vi "Rotate Point.vi"(6 "Para":cluster{"Absolute?":bool, "Angle":dbl}={"Absolute?"=TRUE, "Angle"=0.0}, 8 "错误输入":errorcluster, 10 "Center":T1, 11 "Input Point":T1 caption="Point") -> (0 "错误输出":errorcluster, 2 "Rotated Relative Point":T1 caption="Rotated Relative  Point", 3 "Rotated Absolute Point":T1)   [LabVIEW 2011, in "Basic Shape.lvlib"]
uses:
  Basic Shape.lvlib
  Point Custom Control.ctl
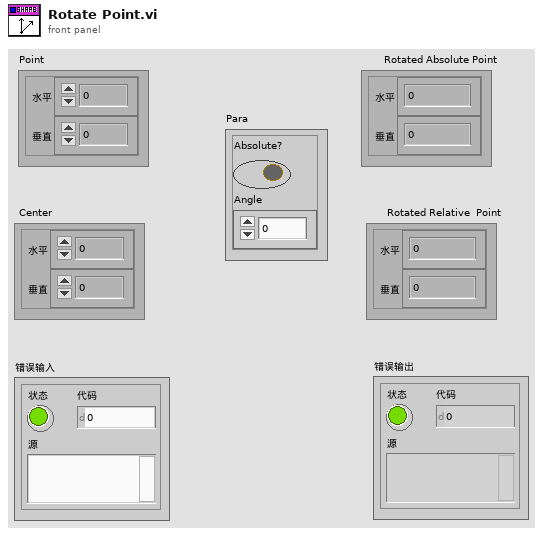
[diagram p1: front panel]
types:
  T1 = typedef "Basic Shape.lvlib/Point Custom Control.ctl" = cluster{"horizontal":i16, "vertical":i16}
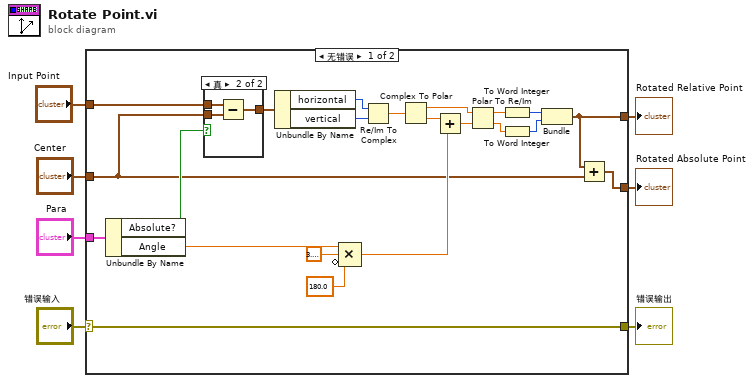
[diagram p0: block diagram]
diagram:
  n1 = case shown="无错误" "错误输入" {
    selector: "错误输入" -> [w9 w35]
    tunnel: [w9 w35] -> w6
    tunnel: "Para" -> [w29 _]
    tunnel: "Input Point" -> [w27 w34]
    tunnel: "Center" -> [w11 _]
    tunnel: [w12 w34] -> w2
    tunnel: [w10 w34] -> w1
    frame No Error {
      n2 = Unbundle By Name(w29) -> ("Absolute?"=w28:bool, "Angle"=w8:dbl)
      n3 = case shown="真" w28 {
        tunnel: w27 -> [w30 w33]
        tunnel: w11 -> [_ w32]
        tunnel: [w30 w31] -> w26
        frame False {
        }
        frame True {
          n4 = Subtract(x=w33, y=w32) -> (x-y=w31:T1)
        }
      }
      n5 = Unbundle By Name(w26) -> ("horizontal"=w25:i16, "vertical"=w24:i16)
      n6 = Compound Arithmetic op=MULTIPLY(w8, 3.141592653589793, invert 180.0 ("值")) -> (w19:dbl)
      n7 = Re/Im To Complex(1:w24, 2:w25) -> (0:w23:cdb)
      n8 = Complex To Polar(r * e^(i*theta)=w23) -> (r=w17:dbl, theta=w20:dbl)
      n9 = Add(x=w20, y=w19) -> (x+y=w18:dbl)
      n10 = Polar To Re/Im(2:w18, 3:w17) -> (0:w15:dbl, 1:w16:dbl)
      n11 = To Word Integer(number=w16) -> (16bit integer=w14:i16)
      n12 = To Word Integer(number=w15) -> (16bit integer=w13:i16)
      n13 = Bundle(w14, w13) -> (w12:cluster{i16, i16})  [unwired: 1 in]
      n14 = Add(x=w12, y=w11) -> (x+y=w10:T1)
    }
    frame Error {
    }
  }
  "错误输出" <- w6
  "Rotated Absolute Point" <- w1
  "Rotated Relative Point" <- w2
